vi "Add Entry.vi"(10 "Object Entry":refnum<class "OD Section.lvclass">, 11 "Object Dictionary in":refnum<class "Object Dictionary.lvclass">) -> (3 "Object Dictionary out":refnum<class "Object Dictionary.lvclass">)   [LabVIEW 2024, in "EDS.lvlib" / "Object Dictionary.lvclass"]
uses:
  Object Dictionary.lvclass
  Object Dictionary.lvclass/Object Dictionary.ctl
  OD Section/OD Section.lvclass
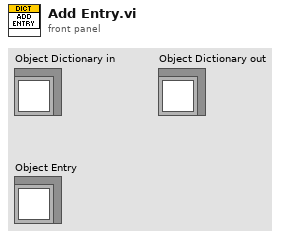
[diagram p1: front panel]
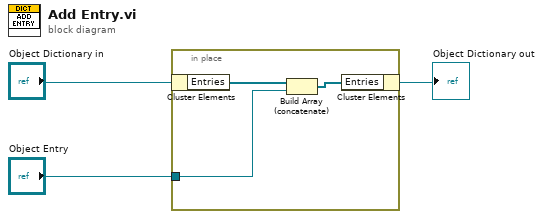
[diagram p0: block diagram]
diagram:
  n1 = in-place {
    in-place-border: "Object Entry" -> [w5]
    n2 = in-place-cluster #1("Object Dictionary in") -> ("Entries"=w6:refnum<class "OD Section.lvclass">[])
    n3 = Build Array (concatenate)(w6, w5) -> (w4:refnum<class "OD Section.lvclass">[])
    n4 = in-place-cluster #1("Entries"=w4) -> (→"Object Dictionary out":refnum<class "Object Dictionary.lvclass">)
  }
